vi "Keithley2100.get interface.vi"(0 "i ref in":refnum<vi>, 5 "error in (no error)":errorcluster) -> (14 "i refout":refnum<vi>, 16 "Interface":string, 19 "error out":errorcluster)   [LabVIEW 2014, in "Keithley2100.lvlib"]
doc: "This VI is used to get the USB port of the USBSwitchBox from the database.\n\nLicense Agreement for this software:\n\nCopyright (C)\nGesellschaft für Schwerionenforschung, GSI\nPlanckstr. 1\n64291 Darmstadt\nGermany\n\nContact: D.Beck@gsi.de \n\nThis program is free software; you can redistribute it and/or modify it under the terms of the \nGNU General Public License as published by the Free Software Foundation; either version 2 of \nthe license, or (at your option) any later version.\n\nThis program is distributed in the hope that it will be useful, but WITHOUT ANY WARRANTY; \nwithout even the implied warranty of MERCHANTABILITY or FITNESS FOR A PARTICULAR PURPOSE. See the GNU General License for more details (http://www.gnu.org).\n\nGesellschaft für Schwerionenforschung, GSI\nPlanckstr. 1, 64291 Darmstadt, Germany\nFor all questions and ideas contact: M.Richter@gsi.de, H.Brand@gsi.de or D.Beck@gsi.de.\nLast update: 16-JUN-2004"
uses:
  Keithley2100.lvlib
  CS_Core/BaseProcess/BaseProcess.lvlib
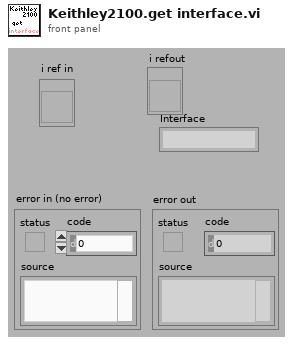
[diagram p1: front panel]
types:
  T1 = typedef "BaseProcess.lvlib/BaseProcess.i attribute.ctl" = cluster{"EventStatus":string, "EventError":i32, "PresetEvtWatchD":i32, "PresetPdcWatchD":i32, "EventTimeout":i32, "PeriodicInterval":i32, "Interface":string[], "Address":string[], "Special":string[], "PeriodicError":i32, "PeriodicStatus":string, "SuperProc":string, "Descriptors":T2[], "CaseRef":refnum<vi>, "PdcRef":refnum<vi>, "Thread Ref":refnum<vi>, "eventErrorID":i32, "eventStatusID":i32, "periodicErrorID":i32, "periodicStatusID":i32, "pdcCtrID":i32}
  T2 = typedef "BaseProcess.lvlib/BaseProcess.descriptor definition.ctl" = cluster{"selector":string, "descriptor":T3}
  T3 = typedef "BaseProcess.lvlib/BaseProcess.descriptor string definition.ctl" = string
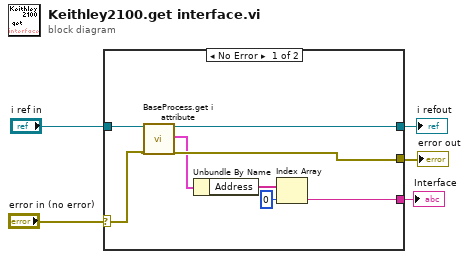
[diagram p0: block diagram]
diagram:
  n1 = case shown="No Error" "error in (no error)" {
    selector: "error in (no error)" -> [w12 w15]
    tunnel: [w10 w15] -> w3
    tunnel: "i ref in" -> [w13 w14]
    tunnel: [w11 w14] -> w2
    tunnel: [w6 _] -> w1
    frame No Error {
      n2 = call "BaseProcess.get i attribute.vi"("i ref in"=w13, "error in (no error)"=w12) -> ("i ref out"=w11:refnum<vi>, "i attribute"=w9:T1, "error out"=w10:errorcluster)  [unwired: 15 in]
      n3 = Unbundle By Name(w9) -> ("Address"=w8:string[])
      n4 = Index Array(array=w8, index=0) -> (element=w6:string)
    }
    frame Error {
    }
  }
  "error out" <- w3
  "i refout" <- w2
  "Interface" <- w1
